vi "Copy CD Built Files.vi"(8 "error in (no error)":errorcluster, 10 "Project XML Editor in":refnum<class "Project XML Editor.lvclass">) -> (0 "error out":errorcluster, 2 "Project XML Editor out":refnum<class "Project XML Editor.lvclass">)   [LabVIEW 2020, in "LVLIBP CD XML Updater.lvlib"]
uses:
  LVLIBP CD XML Updater.lvlib
  Project XML Editor/Project XML Editor.lvclass
  Project XML Editor/Project XML Editor.lvclass/Project XML Editor.ctl
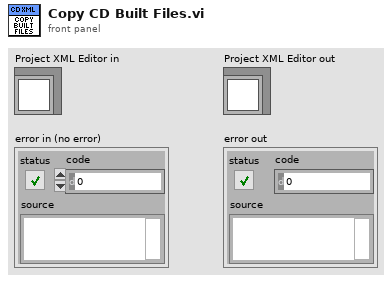
[diagram p1: front panel]
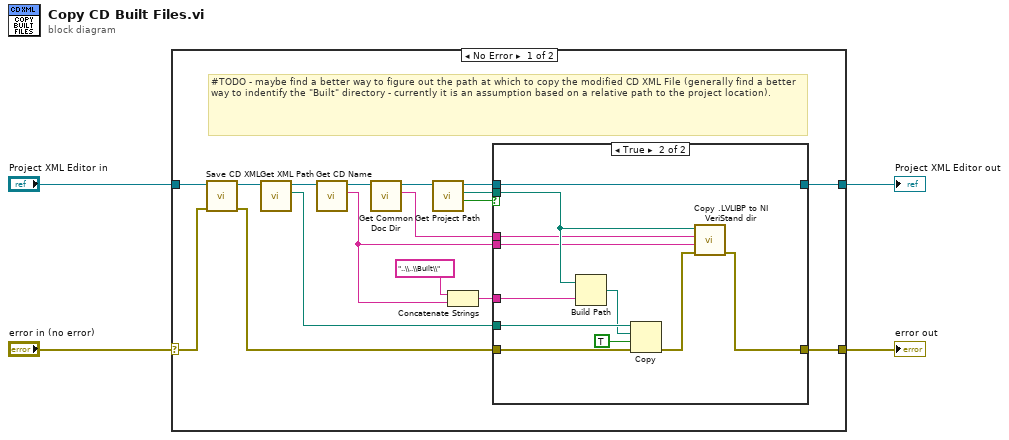
[diagram p0: block diagram]
diagram:
  n1 = case shown="No Error" "error in (no error)" {
    selector: "error in (no error)" -> [w6 w35]
    tunnel: [w9 w36] -> w4
    tunnel: [w21 w35] -> w3
    tunnel: "Project XML Editor in" -> [w8 w36]
    frame No Error {
      # "#TODO - maybe find a better way to figure out the path at which to copy the modified CD XML File (generally find a better way to indentify the \"Built\" directory - currently it is an assumption based on a relative path to the project location)."
      n2 = call "Save CD XML.vi"("error in (no error)"=w6, "Project XML Editor in"=w8) -> ("error out"=w5:errorcluster, "Project XML Editor out"=w7:refnum<class "Project XML Editor.lvclass">)  [unwired: 8 in]
      n3 = call "Get XML Path.vi"("Project XML Editor in"=w7) -> ("XML Path"=w19:path, "Project XML Editor out"=w17:refnum<class "Project XML Editor.lvclass">)  [unwired: 9 in]
      n4 = call "Get CD Name.vi"("Project XML Editor in"=w17) -> ("CD Name"=w18:string, "Project XML Editor out"=w12:refnum<class "Project XML Editor.lvclass">)  [unwired: 9 in]
      n5 = call "Get Common Doc Dir.vi"("Project XML Editor in"=w12) -> ("Common Doc Dir"=w14:string, "Project XML Editor out"=w13:refnum<class "Project XML Editor.lvclass">)  [unwired: 9 in]
      n6 = call "Get Project Path.vi"("Project XML Editor in"=w13) -> ("Available?"=w11:bool, "Source Project Path"=w20:path, "Project XML Editor out"=w10:refnum<class "Project XML Editor.lvclass">)  [unwired: 8 in]
      n7 = Concatenate Strings("..\\..\\Built\\" ("string"), w18) -> (w16:string)
      n8 = case shown="True" w11 {
        tunnel: [w22 w34] -> w21
        tunnel: w20 -> [_ w32]
        tunnel: w19 -> [_ w30]
        tunnel: w18 -> [_ w29]
        tunnel: w16 -> [_ w28]
        tunnel: w14 -> [_ w27]
        tunnel: w5 -> [w22 w26]
        tunnel: w10 -> [w23 w25]
        tunnel: [w23 w25] -> w9
        frame False {
        }
        frame True {
          n9 = Build Path(base path=w32, name or relative path=w28) -> (appended path=w24:path)
          n10 = Copy(8:w26, 9:TRUE ("overwrite (F)"), 10:w24, 11:w30) -> (0:w33:errorcluster)  [unwired: 1 in, 2 out]
          n11 = call "Copy .LVLIBP to NI VeriStand dir.vi"("error in (no error)"=w33, "CD name"=w29, "CD Folder name"=w27, "Project Path"=w32) -> ("error out"=w34:errorcluster)  [unwired: 7 in]
        }
      }
    }
    frame Error {
    }
  }
  "Project XML Editor out" <- w4
  "error out" <- w3
